vi "Get ID.vi"(11 "Plugin in":refnum<class "Plugin.lvclass">) -> (2 "id":i32, 3 "Plugin out":refnum<class "Plugin.lvclass">)   [LabVIEW 2019, in "DSF Core.lvlib" / "Plugin.lvclass"]
uses:
  Plugin.lvclass
  Plugin.lvclass/Plugin.ctl
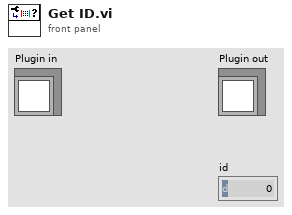
[diagram p1: front panel]
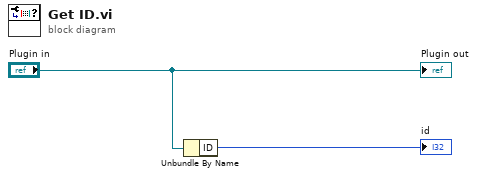
[diagram p0: block diagram]
diagram:
  n1 = Unbundle By Name("Plugin in") -> ("ID"=→"id":i32)
  "Plugin out" <- "Plugin in"
